vi "Matlab_1.vi"(8 "Fehler (Eingang, kein Fehler)":errorcluster, 9 "Subject ID":dbl, 10 "Impactor ID":dbl, 11 "Username":string) -> (0 "Fehler (Ausgang)":errorcluster, 3 "Name":string)   [LabVIEW 2020]
panel:
  out "impactor":bool
  out "user":bool
  out "subject":bool
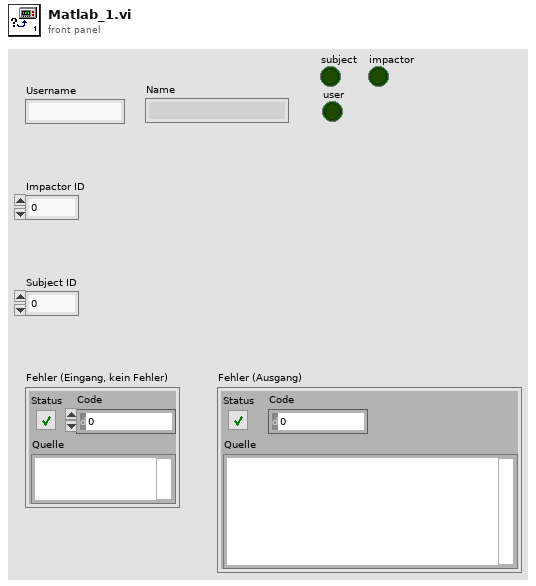
[diagram p1: front panel]
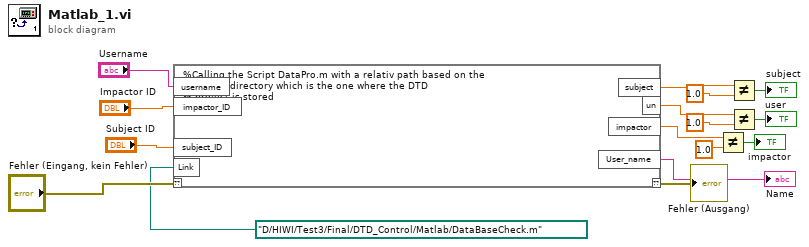
[diagram p0: block diagram]
diagram:
  n1 = script code="%Calling the Script DataPro.m with a relativ path based on the \n%current directory which is the one where the DTD \n% project is stored\nrun(Link)"("??"="Fehler (Eingang, kein Fehler)", "impactor_ID"="Impactor ID", "username"="Username", "subject_ID"="Subject ID", "Link"=path "D:/HIWI/Test3/Final/DTD_Control/Matlab/DataBaseCheck.m" ("Path")) -> ("??"=→"Fehler (Ausgang)":errorcluster, "impactor"=w6:dbl, "un"=w5:dbl, "User_name"=→"Name":string, "subject"=w11:dbl)
  n2 = Not Equal?(x=w6, y=1.0) -> (x != y?=→"impactor":bool)
  n3 = Not Equal?(x=w11, y=1.0) -> (x != y?=→"subject":bool)
  n4 = Not Equal?(x=w5, y=1.0) -> (x != y?=→"user":bool)
